vi "Source Mode query.vi"(8 "error in (no error)":errorcluster, 10 "Step":T1=1 min=1 max=99 step=1, 11 "VISA resource name":refnum<visa-resource-name>) -> (0 "error out":errorcluster, 2 "Mode":string, 3 "VISA resource name out":refnum<visa-resource-name>)   [LabVIEW 2025, in "Chroma 19572.lvlib"]
doc: "Chroma\n5 Clock Tower Place Suite 210\nMaynard, MA 01754\nTel: 1 800 253-1230\nTel: 1 877 4 A HIPOT\nFax: 1 978-461-4295\nWebsite: www.chroma.com"
uses:
  <instrlib>/Chroma 19572/Chroma 19572.lvlib
  <instrlib>/Chroma 19572/Public/Utility/Type Def/steps--numeric.ctl
panel:
  # "MODE by Step query"
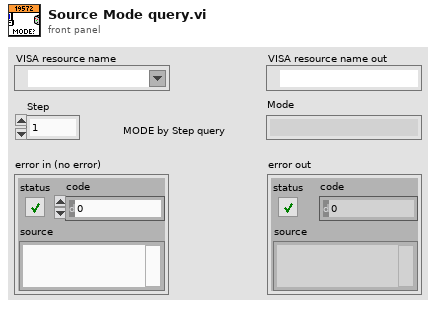
[diagram p1: front panel]
types:
  T1 = typedef "Chroma 19572.lvlib/steps--numeric.ctl" = u8
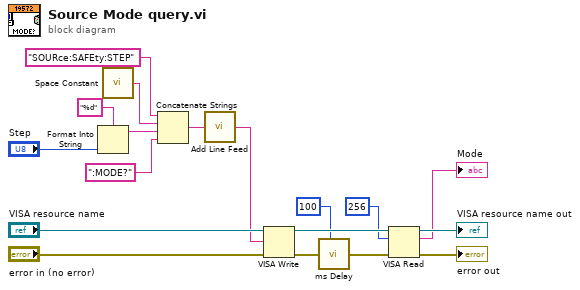
[diagram p0: block diagram]
diagram:
  n1 = Format Into String(format string="%d", "Step") -> (resulting string=w8:string)  [unwired: 2 in, 1 out]
  n2 = call <vilib>:"Space Constant.vi"() -> ("String"=w6:string)
  n3 = Concatenate Strings("SOURce:SAFEty:STEP", w6, w8, ":MODE?") -> (w4:string)
  n4 = call <instrlib>:"Add Line Feed.vi"("Command string"=w4) -> ("Concatenated string"=w14:string)  [unwired: 4 in]
  n5 = VISA Write(VISA resource name="VISA resource name", write buffer=w14, error in (no error)="error in (no error)") -> (VISA resource name out=w18:refnum<visa-resource-name>, error out=w3:errorcluster)  [unwired: 1 out]
  n6 = call <instrlib>:"ms Delay.vi"("miliseconds to wait"=u32 100 ("Time Delay ms"), "error in (no error)"=w3) -> ("error out"=w2:errorcluster)  [unwired: 6 in, 1 out]
  n7 = VISA Read(VISA resource name=w18, byte count=u32 256, error in (no error)=w2) -> (VISA resource name out=→"VISA resource name out":refnum<visa-resource-name>, read buffer=→"Mode":string, error out=→"error out":errorcluster)  [unwired: 1 out]
